vi "Right Rocket Double Level 2.vi"   [LabVIEW 2018]
uses:
  Auton Kill Switch.vi
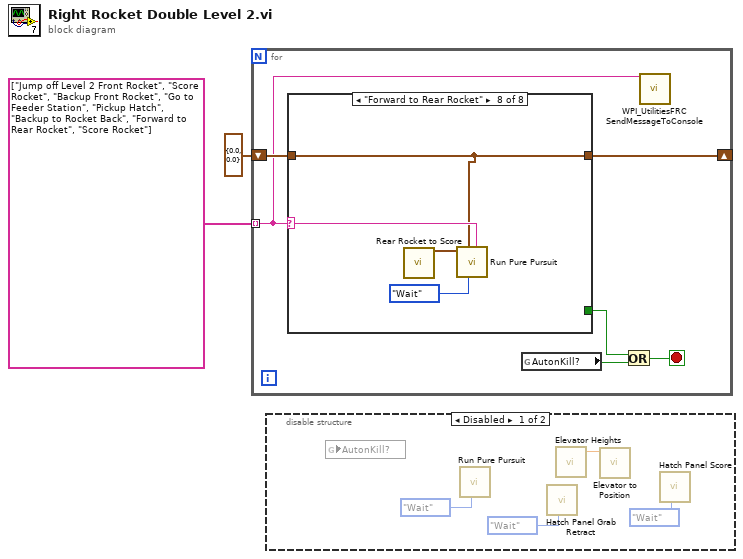
[diagram p0: block diagram]
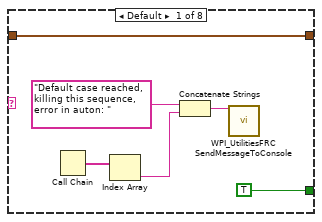
[diagram p3: hidden frame]
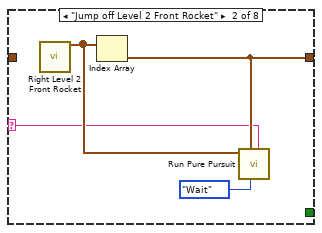
[diagram p4: hidden frame]
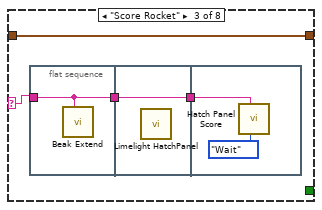
[diagram p5: hidden frame]
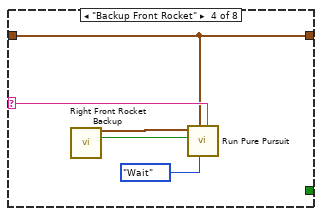
[diagram p6: hidden frame]
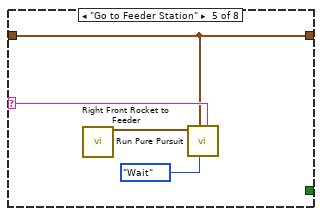
[diagram p7: hidden frame]
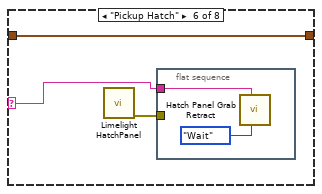
[diagram p8: hidden frame]
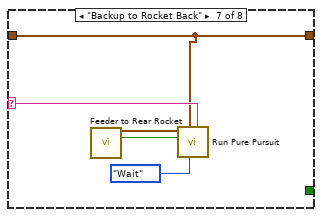
[diagram p9: hidden frame]
diagram:
  n1 = for {
    tunnel: string[] ["Jump off Level 2 Front Rocket", "Score Rocket", "Backup Front Rocket", "Go to Feeder Station", "Pickup Hatch", "Backup to Rocket Back", "Forward to Rear Rocket", "Score Rocket"] -> [w3] mode=indexing
    shift-right: [w7] -> _
    shift-left: cluster{"X":dbl, "Y":dbl} {"X"=0.0, "Y"=0.0} -> [w6]
    stop <- w5 stop-if-true
    n2 = case shown="\"Forward to Rear Rocket\"" w3 {
      selector: w3 -> [_ w15 w21 w28 w34 w36 w44 w48]
      tunnel: [w13 w16 w22 w27 w33 w38 w43 w47] -> w7
      tunnel: w6 -> [w13 _ w22 w27 w33 w38 w43 w47]
      tunnel: [TRUE _ _ _ _ _ _ _] -> w4
      frame Default {
        n3 = Call Chain() -> (call chain=w12:string[])
        n4 = Index Array(array=w12) -> (element=w10:string)  [unwired: 1 in]
        n5 = Concatenate Strings("Default case reached, killing this sequence, error in auton: " ("Message"), w10) -> (w9:string)
        n6 = call <vilib>:"WPI_UtilitiesFRC SendMessageToConsole.vi"("Message"=w9) -> ()  [unwired: 14 in, 1 out]
      }
      frame "Jump off Level 2 Front Rocket" {
        n7 = call "Right Level 2 Front Rocket.vi"() -> ("path"=w17:cluster{"X":dbl, "Y":dbl}[])  [unwired: 15 in]
        n8 = Index Array(array=w17) -> (element=w16:cluster{"X":dbl, "Y":dbl})  [unwired: 1 in]
        n9 = call "Run Pure Pursuit.vi"("Description"=w15, "Synchronication"=enum16{"Start", "Wait"}."Wait", "Auton Start Point"=w16, "Path"=w17) -> ()  [unwired: 7 in, 1 out]
      }
      frame "Score Rocket" {
        n10 = flat-sequence {
          tunnel: w21 -> [w23]
          tunnel: [w23] -> w19
          tunnel: [w24] -> w20
          tunnel: w19 -> [w24]
          tunnel: w20 -> [w25]
          frame #0 {
            n11 = call "Beak Extend.vi"("Description"=w23) -> ()  [unwired: 10 in, 1 out]
          }
          frame #1 {
            n12 = call "Limelight HatchPanel.vi"() -> ()  [unwired: 11 in, 1 out]
          }
          frame #2 {
            n13 = call "Hatch Panel Score.vi"("Synchronization"=enum16{"Start", "Wait"}."Wait", "Description"=w25) -> ()  [unwired: 9 in, 1 out]
          }
        }
      }
      frame "Backup Front Rocket" {
        n14 = call "Right Front Rocket Backup.vi"() -> ("path"=w30:cluster{"X":dbl, "Y":dbl}[], "Reverse Path?"=w29:bool)  [unwired: 14 in]
        n15 = call "Run Pure Pursuit.vi"("Description"=w28, "Synchronication"=enum16{"Start", "Wait"}."Wait", "Auton Start Point"=w27, "Reverse? (F)"=w29, "Path"=w30) -> ()  [unwired: 6 in, 1 out]
      }
      frame "Go to Feeder Station" {
        n16 = call "Right Front Rocket to Feeder.vi"() -> ("path"=w32:cluster{"X":dbl, "Y":dbl}[])  [unwired: 15 in]
        n17 = call "Run Pure Pursuit.vi"("Description"=w34, "Synchronication"=enum16{"Start", "Wait"}."Wait", "Auton Start Point"=w33, "Path"=w32) -> ()  [unwired: 7 in, 1 out]
      }
      frame "Pickup Hatch" {
        n18 = call "Limelight HatchPanel.vi"() -> ("error out"=w37:errorcluster)  [unwired: 11 in]
        n19 = flat-sequence {
          tunnel: w37 -> [_]
          tunnel: w36 -> [w39]
          frame #0 {
            n20 = call "Hatch Panel Grab Retract.vi"("Synchronization"=enum16{"Start", "Wait"}."Wait", "Description"=w39) -> ()  [unwired: 9 in, 1 out]
          }
        }
      }
      frame "Backup to Rocket Back" {
        n21 = call "Feeder to Rear Rocket.vi"() -> ("path"=w42:cluster{"X":dbl, "Y":dbl}[], "Reverse Path?"=w41:bool)  [unwired: 14 in]
        n22 = call "Run Pure Pursuit.vi"("Description"=w44, "Synchronication"=enum16{"Start", "Wait"}."Wait", "Auton Start Point"=w43, "Reverse? (F)"=w41, "Path"=w42) -> ()  [unwired: 6 in, 1 out]
      }
      frame "Forward to Rear Rocket" {
        n23 = call "Rear Rocket to Score.vi"() -> ("path"=w46:cluster{"X":dbl, "Y":dbl}[])  [unwired: 15 in]
        n24 = call "Run Pure Pursuit.vi"("Description"=w48, "Synchronication"=enum16{"Start", "Wait"}."Wait", "Auton Start Point"=w47, "Path"=w46) -> ()  [unwired: 7 in, 1 out]
      }
    }
    n25 = global read "Auton Kill Switch.vi" "AutonKill?"() -> (w8:bool)
    n26 = Or(x=w4, y=w8) -> (x .or. y?=w5:bool)
    n27 = call <vilib>:"WPI_UtilitiesFRC SendMessageToConsole.vi"("Message"=w3) -> ()  [unwired: 14 in, 1 out]
  }
  n28 = disable-structure shown="Disabled" {
    frame Disabled {
      n29 = global read "Auton Kill Switch.vi" "AutonKill?"() -> ()  [unwired: 1 in]
      n30 = call "Run Pure Pursuit.vi"("Synchronication"=enum16{"Start", "Wait"}."Wait") -> ()  [unwired: 10 in, 1 out]
      n31 = call "Hatch Panel Grab Retract.vi"("Synchronization"=enum16{"Start", "Wait"}."Wait") -> ()  [unwired: 10 in, 1 out]
      n32 = call "Elevator Heights.vi"() -> ("Height"=w52:dbl)  [unwired: 9 in, 2 out]
      n33 = call "Elevator to Position.vi"("Elevator Height"=w52) -> ()  [unwired: 10 in, 1 out]
      n34 = call "Hatch Panel Score.vi"("Synchronization"=enum16{"Start", "Wait"}."Wait") -> ()  [unwired: 10 in, 1 out]
    }
    frame Enabled {
    }
  }
